vi "Message Window.vi"(8 "error in (no error)":errorcluster, 11 "Message string":string) -> (0 "error out (no error)":errorcluster)   [LabVIEW 2017]
doc: "Use this template to create a dialog box with event handling."
uses:
  <vilib>/Utility/miscctls.llb/LVPointTypeDef.ctl
  Global Variables/General Globals.vi
panel:
  out "Message":string
  in  "Close":bool
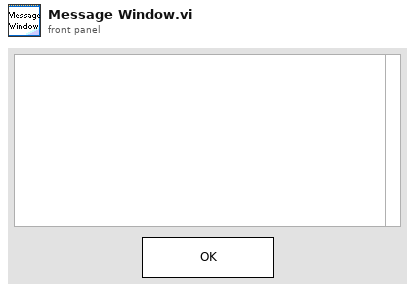
[diagram p1: front panel]
types:
  T1 = typedef "LVPointTypeDef.ctl" = cluster{"Horizontal":i16, "Vertical":i16}
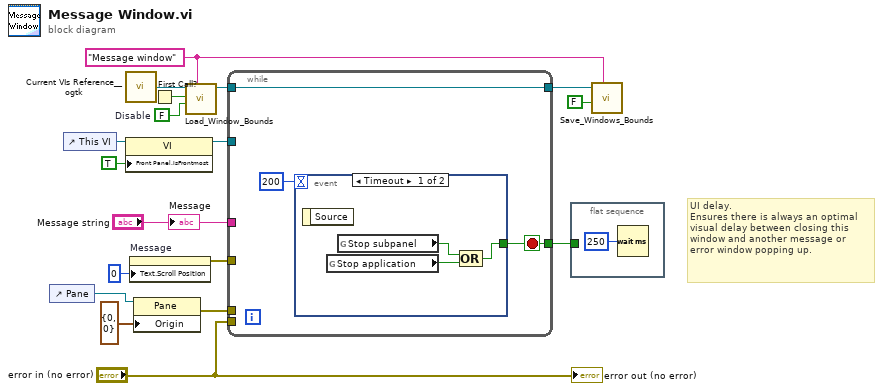
[diagram p0: block diagram]
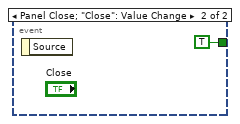
[diagram p2: hidden frame]
diagram:
  w6 = FALSE  # Disable
  w5 = "Message window" ("Window Name (i.e. Key)")
  # "UI delay.\nEnsures there is always an optimal visual delay between closing this window and another message or error window popping up."
  n1 = control-ref of="Pane"() -> (w10:refnum<vi>)
  n2 = control-ref of="This VI"() -> (w14:refnum<vi>)
  n3 = call <userlib>:"Current VIs Reference__ogtk.vi"() -> ("Current VI's reference"=w8:refnum<vi>)  [unwired: 5 in]
  n4 = property on="Property Node" class="VI"(reference=w14, "Front Panel.IsFrontmost"=TRUE ("Front Panel Window:Is Frontmost")) -> (reference out=w13:refnum<vi>)  [unwired: 1 in, 1 out]
  n5 = property on="Message" class="Str"("Text.Scroll Position"=u32 0) -> (error out=w16:errorcluster)  [unwired: 2 in, 1 out]
  n6 = property class="Pane"(reference=w10, "Origin"=T1 {"Horizontal"=0, "Vertical"=0}) -> (error out=w11:errorcluster)  [unwired: 1 in, 1 out]
  n7 = First Call?() -> (First Call?: T/F=w7:bool)
  n8 = call "Load_Window_Bounds.vi"("Window Name (i.e. Key)"=w5, "Disable"=w6, "First Call"=w7, "Window VI's Ref"=w8) -> ("reference out"=w3:refnum<vi>)  [unwired: 4 in, 3 out]
  n9 = while {
    tunnel: "Message string" -> [_]
    tunnel: w16 -> [_]
    tunnel: w11 -> [_]
    tunnel: w13 -> [_]
    tunnel: [w20] -> w9
    tunnel: w3 -> [w19]
    tunnel: [w19] -> w2
    tunnel: "error in (no error)" -> [_]
    stop <- w20 stop-if-true
    n10 = event shown="[0] Timeout" {
      selector: _ -> [_ _]
      dyn-events: _ -> [_ _]
      timeout: 200 -> [_ _]
      tunnel: [w22 TRUE ("Stop?")] -> w20
      event Timeout {
        n11 = event-data() -> ()  [unwired: 1 in, 1 out]
        n12 = global read "General Globals.vi" "Stop application"() -> (w24:bool)
        n13 = global read "General Globals.vi" "Stop subpanel"() -> (w23:bool)
        n14 = Compound Arithmetic op=OR(w23, w24) -> (w22:bool)
      }
      event Panel Close; "Close": Value Change {
        n15 = event-data() -> ()  [unwired: 1 in, 1 out]
      }
    }
  }
  n16 = flat-sequence {
    tunnel: w9 -> [_]
    frame #0 {
      n17 = Wait (ms)(milliseconds to wait=u32 250) -> ()  [unwired: 1 out]
    }
  }
  n18 = call "Save_Windows_Bounds.vi"("Window Name (i.e. Key)"=w5, "Front Panel Window:Open"=FALSE, "Window VI's Ref"=w2) -> ()  [unwired: 8 in, 1 out]
  "Message" <- "Message string"
  "error out (no error)" <- "error in (no error)"
